vi "Trigger-message-handler.vi"(8 "error in (no error)":errorcluster, 11 "Object ref in":T1) -> (0 "error out":errorcluster, 3 "Object ref out":T1)   [LabVIEW 2013, in "SLMControl.lvlib" / "SC-Main.lvclass"]
uses:
  SC-Main.lvclass
  Object-reference.ctl
  SC-Main.lvclass/SC-Main.ctl
  Read Client.vi
  Client/Sources/SC-Client.lvclass
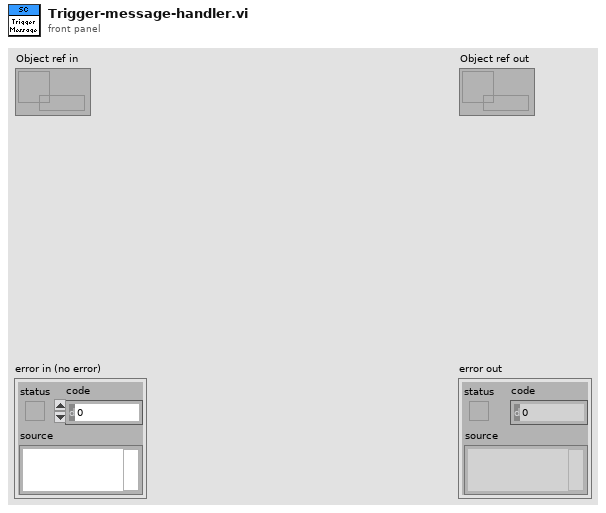
[diagram p1: front panel]
types:
  T1 = typedef "SLMControl.lvlib/SC-Main.lvclass/Object-reference.ctl" = refnum<data-value>
  T2 = typedef "SLMControl.lvlib/SC-Client.lvclass/Object-reference.ctl" = refnum<data-value>
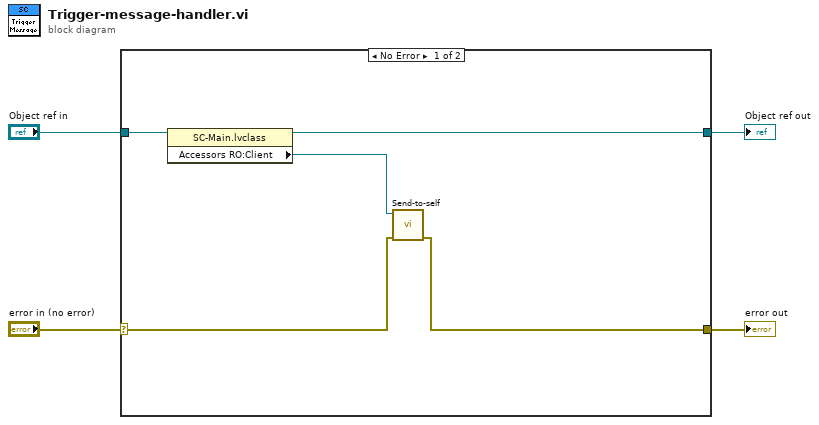
[diagram p0: block diagram]
diagram:
  n1 = case shown="No Error" "error in (no error)" {
    selector: "error in (no error)" -> [w6 w11]
    tunnel: [w5 w11] -> w3
    tunnel: [w8 w10] -> w1
    tunnel: "Object ref in" -> [w9 w10]
    frame No Error {
      n2 = property class="SC-Main.lvclass"(reference=w9) -> (reference out=w8:T1, "Accessors RO:Client"=w7:T2)  [unwired: 1 in, 1 out]
      n3 = call "Send-to-self.vi"("error in (no error)"=w6, "Client in"=w7) -> ("error out"=w5:errorcluster)  [unwired: 8 in, 1 out]
    }
    frame Error {
    }
  }
  "error out" <- w3
  "Object ref out" <- w1
